vi "WriteStdIn.vi"(8 "error in (no error)":errorcluster, 10 "Input":string, 11 ".NET Process in":refnum<class ".NET Process.lvclass">) -> (0 "error out":errorcluster, 3 ".NET Process out":refnum<class ".NET Process.lvclass">)   [LabVIEW 2019, in ".NET Process.lvclass"]
uses:
  .NET Process.lvclass
  .NET Process.lvclass/.NET Process.ctl
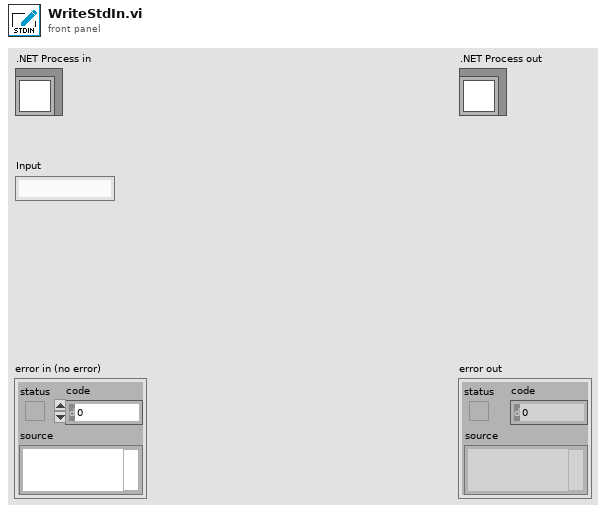
[diagram p1: front panel]
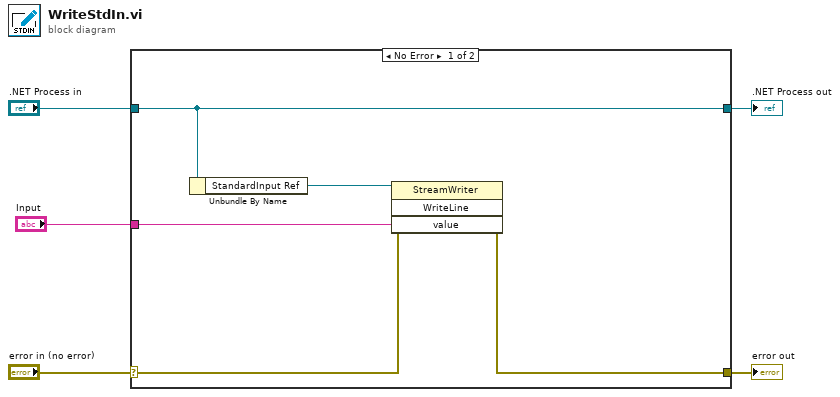
[diagram p0: block diagram]
diagram:
  n1 = case shown="No Error" "error in (no error)" {
    selector: "error in (no error)" -> [w8 w12]
    tunnel: [w7 w12] -> w4
    tunnel: [w10 w11] -> w2
    tunnel: ".NET Process in" -> [w10 w11]
    tunnel: "Input" -> [w6 _]
    frame No Error {
      n2 = Unbundle By Name(w10) -> ("StandardInput Ref"=w9:refnum<k24>)
      n3 = invoke class="StreamWriter" method="WriteLine"(reference=w9, error in=w8, "value"=w6) -> (error out=w7:errorcluster)  [unwired: 1 in, 3 out]
    }
    frame Error {
    }
  }
  "error out" <- w4
  ".NET Process out" <- w2
